vi "Autonomous Independent.vi"() -> ()   [LabVIEW 2014]
doc: "This VI is called when autonomous begins, and will automatically be terminated when autonomous ends. You can carry out timed or sensor driven robot movement independently without needing to return to the caller."
uses:
  <vilib>/Rock Robotics/WPI/Joystick/WPI_JoystickGetSetRefNum.vi
  Robot Global Data.vi
  Events.vi
  <vilib>/Rock Robotics/WPI/RobotDrive/WPI_RobotDriveArcadeDrive_Standard(NoSaturation).vi
panel:
  out "Current Movement, for debugging":T1 {"Y Joystick Value" scale=1.0..-1.0; "X Joystick Value" scale=-1.0..1.0}
  in  "Array of robot movements":T2(array[cluster]) {"Y Joystick Value" scale=1.0..-1.0; "X Joystick Value" scale=-1.0..1.0}
  # "Be sure to right-click and choose Data Operations>>Make Current Value default if you want to save the array values with the VI"
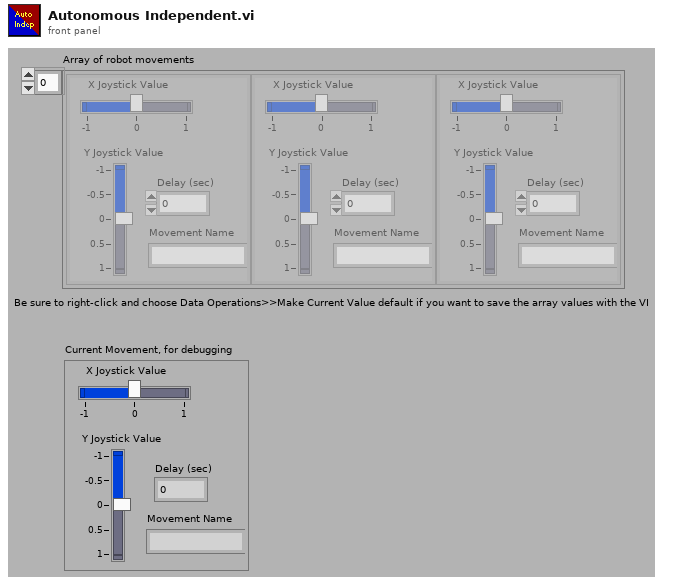
[diagram p1: front panel]
types:
  T1 = cluster{"X Joystick Value":dbl, "Y Joystick Value":dbl, "Delay (sec)":dbl, "Movement Name":string}
  T2 = cluster{"X Joystick Value":dbl, "Y Joystick Value":dbl, "Delay (sec)":dbl, "Movement Name":string}[]
  T3 = typedef "WPI_JoystickDevRef.ctl" = cluster{"Device":T4}
  T4 = typedef "WPI_JoystickDeviceEnum.ctl" = enum16{"USB 0", "USB 1", "USB 2", "USB 3", "USB 4", "USB 5"}
  T5 = cluster{"axis 1 (x)":dbl, "axis 2 (y)":dbl, "axis 3 (throttle)":dbl, "axis 4":dbl, "axis 5":dbl, "axis 6":dbl}
  T6 = typedef "WPI_RobotDriveDevRef.ctl" = cluster{"DevStatus":errorcluster, "Motors[]":T7[], "Square Inputs":bool, "Max Output":dbl}
  T7 = typedef "WPI_MotorControlDeviceRef.ctl" = cluster{"DeviceStatus":errorcluster, "Type":enum16{"PWM", "CAN"}, "PWM":cluster{"Digital Module":T8, "PWM Channel":T9, "DeadBand":T10}, "CAN":cluster{"Device Number":u8, "Control Mode":T11, "Semaphore":T12, "Max Vout":dbl}, "Invert":bool, "TransformRef":T13, "InvTransformRef":T13}
  T8 = typedef "FPGA_TypedefDigitalModule.ctl" = enum16{"Digital Module 1", "Digital Module 2"}
  T9 = typedef "FPGA_DIOPWMChannel.ctl" = enum8{"PWM 1", "PWM 2", "PWM 3", "PWM 4", "PWM 5", "PWM 6", "PWM 7", "PWM 8", "PWM 9", "PWM 10", "Invalid"}
  T10 = typedef "WPI_PWMDeadband.ctl" = cluster{"Name":string, "maxPositivePwm":i32, "minPositivePwm":i32, "centerPwm":i32, "maxNegativePwm":i32, "minNegativePwm":i32, "angularRange":u16}
  T11 = typedef "WPI_CANJaguar_ControlMode.ctl" = enum8{"Percent VBus", "Current", "Speed", "Position", "Voltage"}
  T12 = typedef "Semaphore RefNum" = refnum<k1>
  T13 = typedef "WPI_PWMTransform_ConPane.ctl" = refnum<vi>
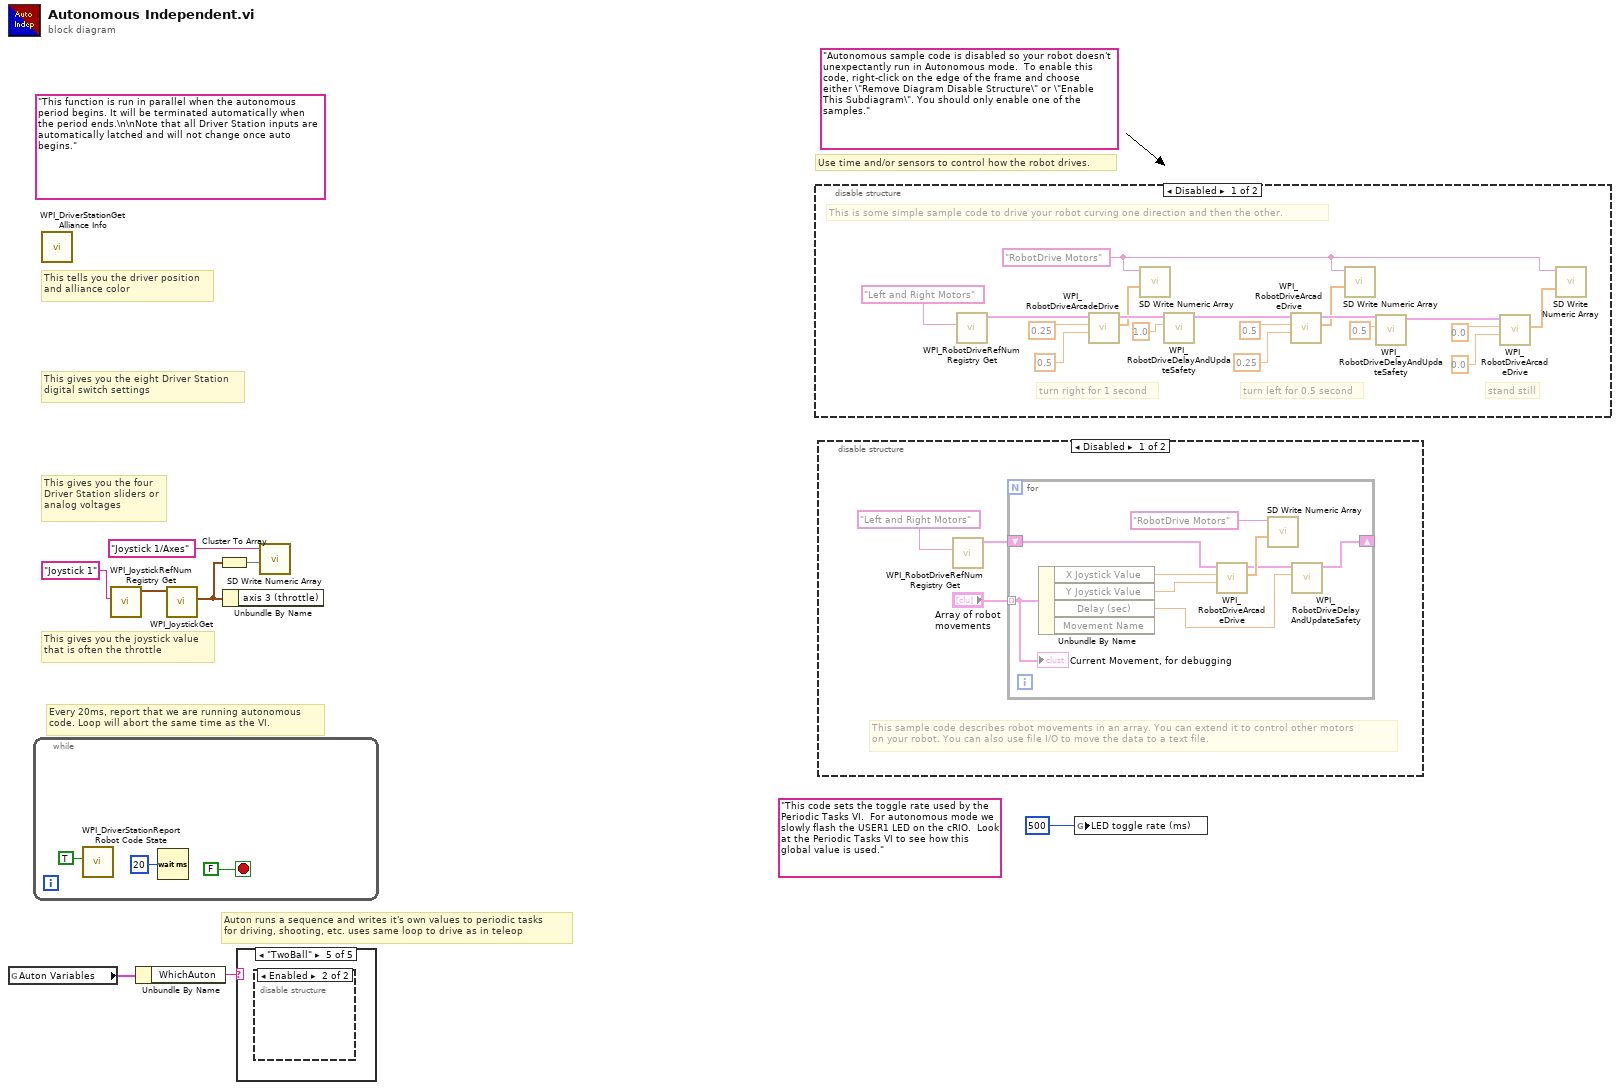
[diagram p0: block diagram]
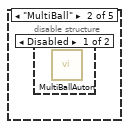
[diagram p3: hidden frame]
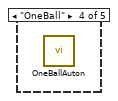
[diagram p6: hidden frame]
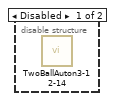
[diagram p7: hidden frame]
diagram:
  (unwired) "This code sets the toggle rate used by the Periodic Tasks VI.  For autonomous mode we slowly flash the USER1 LED on the cRIO.  Look at the Periodic Tasks VI to see how this global value is used."
  (unwired) "Autonomous sample code is disabled so your robot doesn't unexpectantly run in Autonomous mode.  To enable this code, right-click on the edge of the frame and choose either \"Remove Diagram Disable Structure\" or \"Enable This Subdiagram\". You should only enable one of the samples."
  (unwired) "This function is run in parallel when the autonomous period begins. It will be terminated automatically when the period ends.\n\nNote that all Driver Station inputs are automatically latched and will not change once auto begins."
  # "Auton runs a sequence and writes it's own values to periodic tasks\nfor driving, shooting, etc. uses same loop to drive as in teleop"
  # "Every 20ms, report that we are running autonomous\ncode. Loop will abort the same time as the VI."
  # "This gives you the joystick value\nthat is often the throttle"
  # "Use time and/or sensors to control how the robot drives."
  # "This tells you the driver position\nand alliance color"
  # "This gives you the eight Driver Station\ndigital switch settings"
  # "This gives you the four\nDriver Station sliders or\nanalog voltages"
  n1 = global read "Events.vi" "Auton Variables"() -> (w1:cluster{"Hot?":bool, "WhichAuton":string})
  n2 = while {
    stop <- FALSE stop-if-true
    n3 = call <vilib>:"WPI_DriverStationReport Robot Code State.vi"("Autonomous"=TRUE) -> ()  [unwired: 10 in, 1 out]
    n4 = Wait (ms)(milliseconds to wait=u32 20) -> ()  [unwired: 1 out]
  }
  n5 = call <vilib>:"WPI_DriverStationGet Alliance Info.vi"() -> ()  [unwired: 12 out]
  n6 = call <vilib>:"WPI_JoystickRefNum Registry Get.vi"("refnum name"="Joystick 1") -> ("JoystickDevRef"=w7:T3)  [unwired: 1 in, 9 out]
  n7 = Unbundle By Name(w1) -> ("WhichAuton"=w2:string)
  n8 = call <vilib>:"WPI_JoystickGet.vi"("JoystickDevRef"=w7) -> ("Axes"=w4:T5)  [unwired: 1 in, 5 out]
  n9 = Cluster To Array(cluster=w4) -> (array=w5:dbl[])
  n10 = Unbundle By Name(w4) -> ()  [unwired: 1 out]
  n11 = case shown="\"TwoBall\"" w2 {
    frame "BallChase" {
      # "No More Ball Chase\n\n:D\nTROLLL"
    }
    frame "MultiBall" {
      n12 = disable-structure shown="Disabled" {
        frame Disabled {
          n13 = call "MultiBallAuton.vi"() -> ()  [unwired: 12 in]
        }
        frame Enabled {
        }
      }
    }
    frame "none", Default {
    }
    frame "OneBall" {
      n14 = call "OneBallAuton.vi"() -> ()  [unwired: 11 in]
    }
    frame "TwoBall" {
      n15 = disable-structure shown="Enabled" {
        frame Disabled {
          n16 = call "TwoBallAuton3-12-14.vi"() -> ()  [unwired: 12 in]
        }
        frame Enabled {
        }
      }
    }
  }
  n17 = call <vilib>:"SD Write Numeric Array.vi"("Numeric Array"=w5, "Name"="Joystick 1/Axes") -> ()  [unwired: 8 in, 2 out]
  n18 = disable-structure shown="Disabled" {
    frame Disabled {
      w12 = "RobotDrive Motors" ("Name")
      # "This is some simple sample code to drive your robot curving one direction and then the other."
      # "stand still"
      # "turn left for 0.5 second"
      # "turn right for 1 second"
      n19 = call <vilib>:"WPI_RobotDriveRefNum Registry Get.vi"("refnum name"="Left and Right Motors") -> ("RobotDriveDevRef"=w16:T6)  [unwired: 1 in, 9 out]
      n20 = call-poly <vilib>:"WPI_RobotDriveArcadeDrive.vi"("Y axis value"=0.5 ("X axis value"), "X axis value"=0.25, "RobotDriveDevRef"=w16) -> ("Motor Values"=w15:dbl[], "RobotDriveDevRef"=w23:T6)  [unwired: 1 in, 6 out]
      n21 = call <vilib>:"SD Write Numeric Array.vi"("Numeric Array"=w15, "Name"=w12) -> ()  [unwired: 8 in, 2 out]
      n22 = call <vilib>:"WPI_RobotDriveDelayAndUpdateSafety.vi"("Delay (s)"=1.0, "RobotDriveDevRef"=w23) -> ("RobotDriveDevRef 2"=w22:T6)  [unwired: 8 in, 1 out]
      n23 = call-poly <vilib>:"WPI_RobotDriveArcadeDrive.vi"("Y axis value"=0.25 ("X axis value"), "X axis value"=0.5, "RobotDriveDevRef"=w22) -> ("Motor Values"=w14:dbl[], "RobotDriveDevRef"=w21:T6)  [unwired: 1 in, 6 out]
      n24 = call <vilib>:"SD Write Numeric Array.vi"("Numeric Array"=w14, "Name"=w12) -> ()  [unwired: 8 in, 2 out]
      n25 = call <vilib>:"WPI_RobotDriveDelayAndUpdateSafety.vi"("Delay (s)"=0.5, "RobotDriveDevRef"=w21) -> ("RobotDriveDevRef 2"=w20:T6)  [unwired: 8 in, 1 out]
      n26 = call-poly <vilib>:"WPI_RobotDriveArcadeDrive.vi"("Y axis value"=0.0 ("X axis value"), "X axis value"=0.0, "RobotDriveDevRef"=w20) -> ("Motor Values"=w13:dbl[])  [unwired: 1 in, 7 out]
      n27 = call <vilib>:"SD Write Numeric Array.vi"("Numeric Array"=w13, "Name"=w12) -> ()  [unwired: 8 in, 2 out]
    }
    frame Enabled {
    }
  }
  n28 = disable-structure shown="Disabled" {
    frame Disabled {
      # "This sample code describes robot movements in an array. You can extend it to control other motors\non your robot. You can also use file I/O to move the data to a text file."
      n29 = call <vilib>:"WPI_RobotDriveRefNum Registry Get.vi"("refnum name"="Left and Right Motors") -> ("RobotDriveDevRef"=w31:T6)  [unwired: 1 in, 9 out]
      n30 = for {
        shift-right: [w37] -> _
        shift-left: w31 -> [w38]
        tunnel: "Array of robot movements" -> [w33] mode=indexing
        n31 = Unbundle By Name(w33) -> ("X Joystick Value"=w36:dbl, "Y Joystick Value"=w35:dbl, "Delay (sec)"=w34:dbl)  [unwired: 1 out]
        n32 = call-poly <vilib>:"WPI_RobotDriveArcadeDrive.vi"("Y axis value"=w35, "X axis value"=w36, "RobotDriveDevRef"=w38) -> ("Motor Values"=w40:dbl[], "RobotDriveDevRef"=w39:T6)  [unwired: 1 in, 6 out]
        n33 = call <vilib>:"SD Write Numeric Array.vi"("Numeric Array"=w40, "Name"="RobotDrive Motors") -> ()  [unwired: 8 in, 2 out]
        n34 = call <vilib>:"WPI_RobotDriveDelayAndUpdateSafety.vi"("Delay (s)"=w34, "RobotDriveDevRef"=w39) -> ("RobotDriveDevRef 2"=w37:T6)  [unwired: 8 in, 1 out]
        "Current Movement, for debugging" <- w33
      }
    }
    frame Enabled {
    }
  }
  n35 = global write "Robot Global Data.vi" "LED toggle rate (ms)"(u32 500 ("LED ms toggle rate")) -> ()
